vi "convert_boolean_command.vi"(8 "error in (no error)":errorcluster, 11 "Instrument Command":string=":test: ;") -> (0 "error out":errorcluster, 2 "DisableString":string, 3 "EnableString":string)   [LabVIEW 2018]
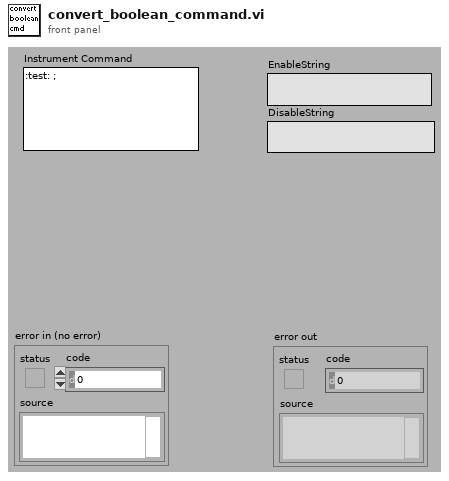
[diagram p1: front panel]
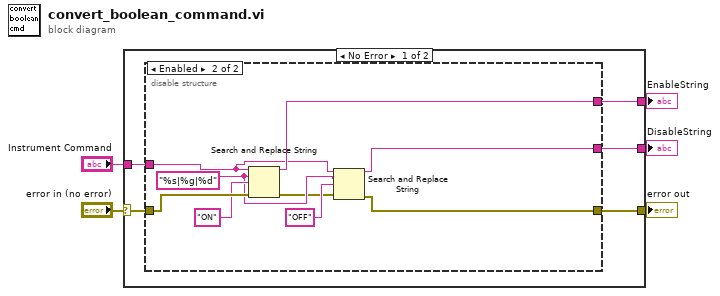
[diagram p0: block diagram]
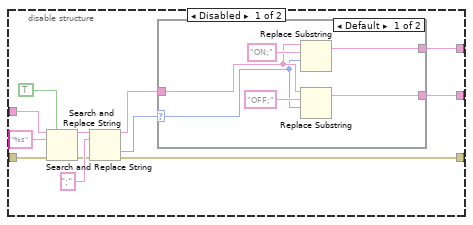
[diagram p2: hidden frame]
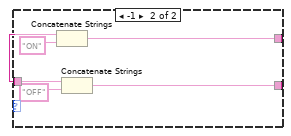
[diagram p3: hidden frame]
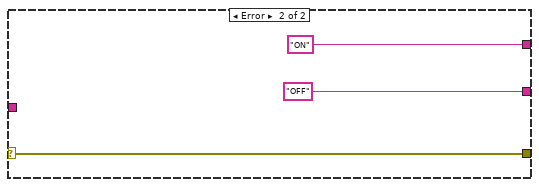
[diagram p4: hidden frame]
diagram:
  n1 = case shown="No Error" "error in (no error)" {
    selector: "error in (no error)" -> [w7 w45]
    tunnel: "Instrument Command" -> [w8 _]
    tunnel: [w10 "ON" ("result string")] -> w4
    tunnel: [w9 "OFF" ("result string")] -> w3
    tunnel: [w6 w45] -> w1
    frame No Error {
      n2 = disable-structure shown="Enabled" {
        disable-tunnel: [w20 w40] -> w10
        disable-tunnel: [w19 w34] -> w9
        disable-tunnel: w8 -> [w17 w39]
        disable-tunnel: w7 -> [w13 w42]
        disable-tunnel: [w11 w35] -> w6
        frame Disabled {
          n3 = Search and Replace String(replace all?=TRUE ("replace all? (F)"), input string=w17, search string="%s", error in=w13) -> (result string=w14:string, error out=w12:errorcluster)  [unwired: 6 out]
          n4 = Search and Replace String(input string=w14, search string=";", error in=w12) -> (result string=w18:string, offset past replacement=w21:i32, error out=w11:errorcluster)  [unwired: 6 out]
          n5 = case shown="Default" w21 {
            selector: w21 -> [w25 _]
            tunnel: w18 -> [w27 w32]
            tunnel: [w24 w30] -> w20
            tunnel: [w23 w29] -> w19
            frame Default {
              n6 = Replace Substring(3:w25, 4:"ON;" ("substring (\"\")"), 5:w27) -> (1:w24:string)  [unwired: 2 out]
              n7 = Replace Substring(3:w25, 4:"OFF;" ("substring (\"\")"), 5:w27) -> (1:w23:string)  [unwired: 2 out]
            }
            frame -1 {
              n8 = Concatenate Strings(w32, "ON" ("string")) -> (w30:string)
              n9 = Concatenate Strings(w32, "OFF" ("string")) -> (w29:string)
            }
          }
        }
        frame Enabled {
          w38 = "%s|%g|%d" ("search string")
          n10 = Search and Replace String(input string=w39, search string=w38, replace string="ON" ("replace string (\"\")"), error in=w42) -> (result string=w40:string, error out=w36:errorcluster)  [unwired: 6 out]
          n11 = Search and Replace String(input string=w39, search string=w38, replace string="OFF" ("replace string (\"\")"), error in=w36) -> (result string=w34:string, error out=w35:errorcluster)  [unwired: 6 out]
        }
      }
    }
    frame Error {
    }
  }
  "EnableString" <- w4
  "DisableString" <- w3
  "error out" <- w1
